vi "Set Skip.vi"(8 "error in (no error)":errorcluster, 10 "Step In":refnum<k7>, 11 "QPA Measurement in":refnum<class "QPA Measurement.lvclass">) -> (0 "error out":errorcluster, 2 "Step Out":refnum<k7>, 3 "QPA Measurement out":refnum<class "QPA Measurement.lvclass">)   [LabVIEW 2016, in "QPA Measurement.lvlib" / "QPA Measurement.lvclass"]
uses:
  QPA Measurement.lvclass
  C:/Projects/STS/Common/Sequence Automation/Plugins/Measurement Interface.lvlibp/Measurement Interface.lvclass
  Plugins/TestStand API Tools (TSAT).lvlibp/Step Actions/Includes/Controls/Run Mode Enum.ctl
  Plugins/Measurement Interface.lvlibp/Private Methods/Measurement Parameters/Read Measurement Parameters.vi
  Plugins/String Database.lvlibp/String Database.lvclass
  Plugins/TestStand API Tools (TSAT).lvlibp/Step Actions/TSAT Step Actions.lvlib
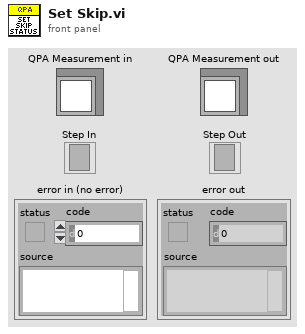
[diagram p1: front panel]
types:
  T1 = typedef "TestStand API Tools (TSAT).lvlibp/TSAT Step Actions.lvlib/Run Mode Enum.ctl" = enum16{"Normal", "Skip", "ForcePass", "ForceFail"}
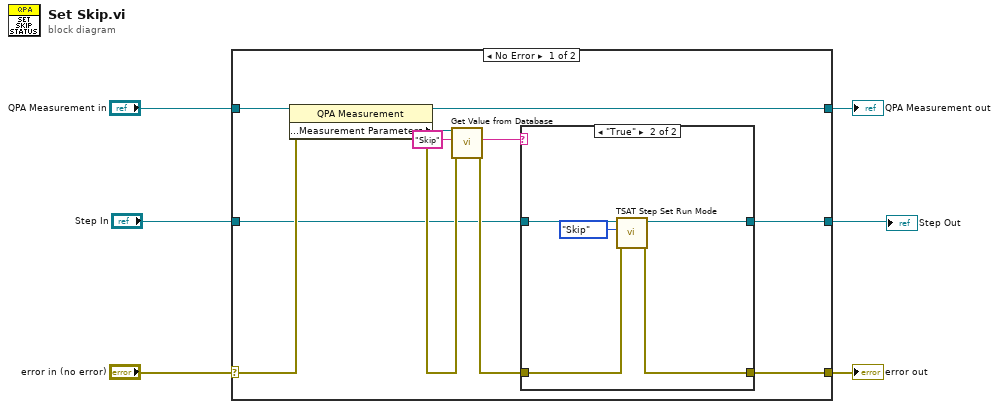
[diagram p0: block diagram]
diagram:
  n1 = case shown="No Error" "error in (no error)" {
    selector: "error in (no error)" -> [w17 w27]
    tunnel: [w9 w27] -> w5
    tunnel: [w15 w26] -> w3
    tunnel: "QPA Measurement in" -> [w16 w26]
    tunnel: "Step In" -> [w8 w25]
    tunnel: [w7 w25] -> w1
    frame No Error {
      n2 = property class="QPA Measurement"(reference=w16, error in=w17) -> (reference out=w15:refnum<class "QPA Measurement.lvclass">, error out=w12:errorcluster, "Protected Methods:Measurement Parameters"=w14:refnum<class "String Database.lvclass">)
      n3 = call "Get Value from Database.vi"("error in (no error)"=w12, "Entry Name"="Skip", "Message in"=w14) -> ("error out"=w10:errorcluster, "Entry Value"=w11:string)  [unwired: 5 in, 2 out]
      n4 = case shown="\"True\"" w11 {
        tunnel: w10 -> [w18 w23]
        tunnel: [w18 w22] -> w9
        tunnel: w8 -> [w19 w21]
        tunnel: [w19 w20] -> w7
        frame "False", Default {
        }
        frame "True" {
          n5 = call "TSAT Step Set Run Mode.vi"("Error In"=w23, "Run Mode"=Run_Mode_Enum."Skip", "Step In"=w21) -> ("Error Out"=w22:errorcluster, "Step Out"=w20:refnum<k7>)  [unwired: 7 in]
        }
      }
    }
    frame Error {
    }
  }
  "error out" <- w5
  "QPA Measurement out" <- w3
  "Step Out" <- w1
